vi "CompareFace.vi"(7 "tolerance":dbl=0.6, 8 "error in (no error)":errorcluster, 9 "faceEncodingToCheck":refnum<k24>, 10 "knownFaceEncoding":refnum<k24>, 11 "FaceRecognition in":refnum<class "FaceRecognition.lvclass">) -> (0 "error out":errorcluster, 2 "CompareFace":bool, 3 "FaceRecognition out":refnum<class "FaceRecognition.lvclass">)   [LabVIEW 2020, in "FaceRecognitionDotNet.lvlib" / "FaceRecognition.lvclass"]
uses:
  FaceRecognition.lvclass
  dll/FaceRecognitionDotNet.dll
  FaceRecognition.lvclass/FaceRecognition.ctl
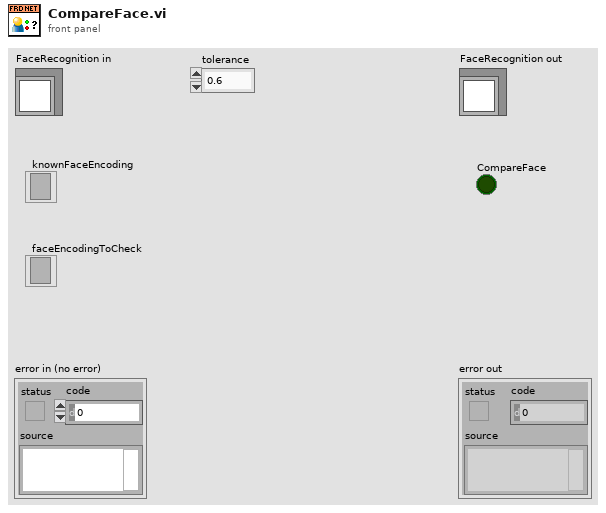
[diagram p1: front panel]
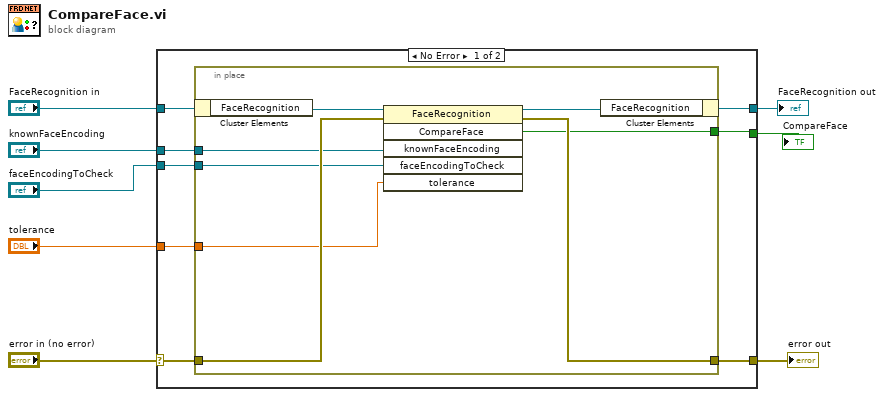
[diagram p0: block diagram]
diagram:
  n1 = case shown="No Error" "error in (no error)" {
    selector: "error in (no error)" -> [w14 w26]
    tunnel: [w13 w26] -> w7
    tunnel: [w15 w25] -> w5
    tunnel: "FaceRecognition in" -> [w16 w25]
    tunnel: [w12 _] -> w4
    tunnel: "knownFaceEncoding" -> [w11 _]
    tunnel: "faceEncodingToCheck" -> [w10 _]
    tunnel: "tolerance" -> [w9 _]
    frame No Error {
      n2 = in-place {
        in-place-border: w14 -> [w22]
        in-place-border: [w21] -> w13
        in-place-border: [w20] -> w12
        in-place-border: w11 -> [w19]
        in-place-border: w10 -> [w18]
        in-place-border: w9 -> [w17]
        n3 = in-place-cluster #1(w16) -> ("FaceRecognition"=w24:refnum<k24>)
        n4 = invoke class="FaceRecognition" method="CompareFace"(reference=w24, error in=w22, "knownFaceEncoding"=w19, "faceEncodingToCheck"=w18, "tolerance"=w17) -> (reference out=w23:refnum<k24>, error out=w21:errorcluster, "CompareFace"=w20:bool)  [unwired: 1 in, 3 out]
        n5 = in-place-cluster #1("FaceRecognition"=w23) -> (w15:refnum<class "FaceRecognition.lvclass">)
      }
    }
    frame Error {
    }
  }
  "error out" <- w7
  "FaceRecognition out" <- w5
  "CompareFace" <- w4
